vi "依行或列索引2D数组(TimeStamp).vi"(8 "error in (no error)":errorcluster caption="错误输入（无错误）", 9 "选择行列":enum16{"行", "列"}(ring), 10 "索引":i32[](array[numeric]), 11 "输入数组":timestamp[][](array[timestamp])) -> (0 "error out":errorcluster caption="错误输出", 3 "元素":timestamp[][](array[timestamp]))   [LabVIEW 2012]
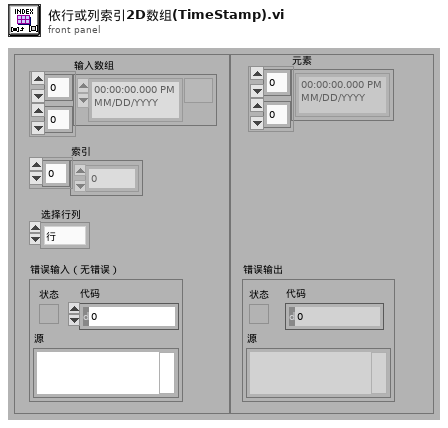
[diagram p1: front panel]
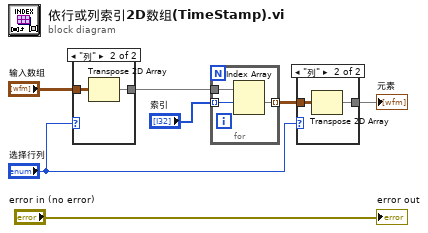
[diagram p0: block diagram]
diagram:
  n1 = case shown="\"列\"" "选择行列" {
    tunnel: [w8 w9] -> w5
    tunnel: "输入数组" -> [w8 w10]
    frame "行", Default {
    }
    frame "列" {
      n2 = Transpose 2D Array(2D array=w10) -> (transposed array=w9:timestamp[][])
    }
  }
  n3 = for {
    tunnel: "索引" -> [w11] mode=indexing
    tunnel: w5 -> [w13]
    tunnel: [w12] -> w2 mode=indexing
    n4 = Index Array(array=w13, index (row)=w11) -> (element=w12:timestamp[])  [unwired: 1 in]
  }
  n5 = case shown="\"列\"" "选择行列" {
    tunnel: w2 -> [w14 w16]
    tunnel: [w14 w15] -> w1
    frame "行", Default {
    }
    frame "列" {
      n6 = Transpose 2D Array(2D array=w16) -> (transposed array=w15:timestamp[][])
    }
  }
  "元素" <- w1
  "error out" <- "error in (no error)"
